vi "Play.vi"(8 "error in (no error)":errorcluster, 11 "Match in":refnum<class "Match.lvclass">) -> (0 "error out":errorcluster, 3 "Match out":refnum<class "Match.lvclass">)   [LabVIEW 2016, in "Match.lvclass"]
uses:
  Match.lvclass
  Match.lvclass/Match.ctl
  Player/Player.lvclass/Player.ctl
  Player/Player.lvclass
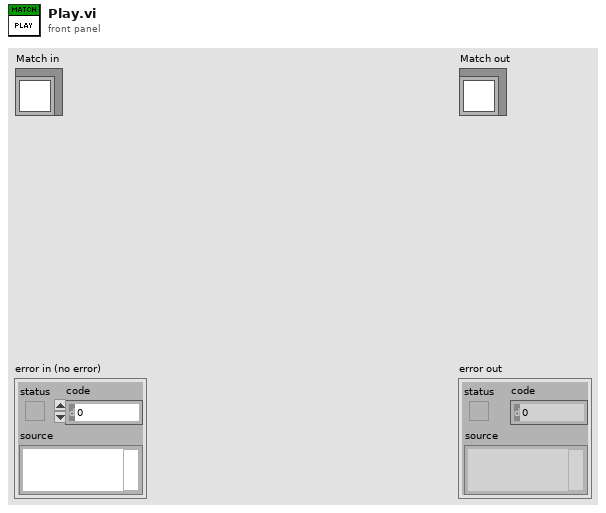
[diagram p1: front panel]
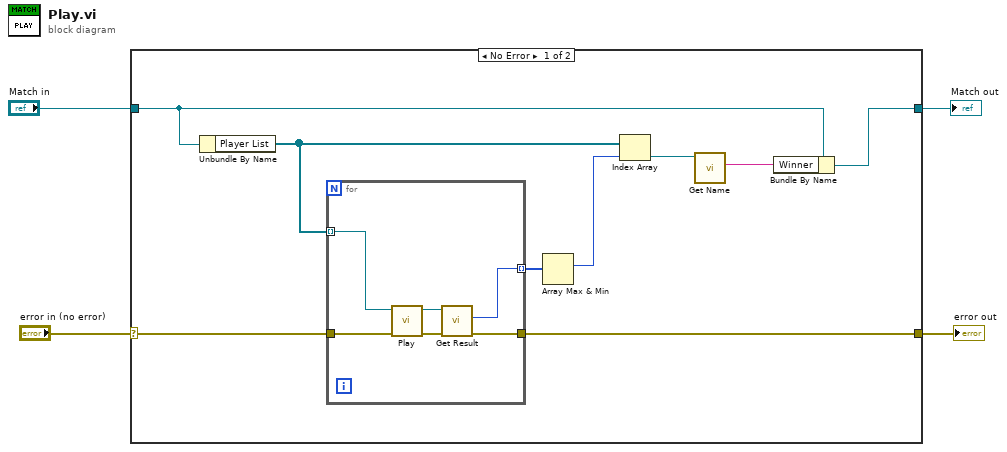
[diagram p0: block diagram]
diagram:
  n1 = case shown="No Error" "error in (no error)" {
    selector: "error in (no error)" -> [w13 w21]
    tunnel: [w12 w21] -> w3
    tunnel: [w5 w20] -> w1
    tunnel: "Match in" -> [w7 w20]
    frame No Error {
      n2 = Unbundle By Name(w7) -> ("Player List"=w10:refnum<class "Player.lvclass">[])
      n3 = for {
        tunnel: w10 -> [w14] mode=indexing
        tunnel: w13 -> [w19]
        tunnel: [w17] -> w12
        tunnel: [w15] -> w11 mode=indexing
        n4 = call "Play.vi"("error in (no error)"=w19, "Player in"=w14) -> ("error out"=w18:errorcluster, "Player out"=w16:refnum<class "Player.lvclass">)  [unwired: 8 in]
        n5 = call "Get Result.vi"("error in (no error)"=w18, "Player in"=w16) -> ("error out"=w17:errorcluster, "Result"=w15:u8)  [unwired: 7 in, 1 out]
      }
      n6 = Array Max & Min(array=w11) -> (max index (indices)=w9:i32)  [unwired: 3 out]
      n7 = Index Array(array=w10, index=w9) -> (element=w8:refnum<class "Player.lvclass">)
      n8 = call "Get Name.vi"("Player in"=w8) -> ("Name"=w6:string)  [unwired: 8 in, 2 out]
      n9 = Bundle By Name(cluster=w7, "Winner"=w6) -> (w5:refnum<class "Match.lvclass">)
    }
    frame Error {
    }
  }
  "error out" <- w3
  "Match out" <- w1
